vi "Set Actuator Voltage.vi"(6 "Enable":variant, 8 "error in (no error)":errorcluster, 9 "AO IOName Idx":i32, 10 "ActuatorV":dbl, 11 "DAQ":refnum<class "DAQ.lvclass">) -> (0 "error out":errorcluster, 3 "DAQ":refnum<class "DAQ.lvclass">)   [LabVIEW 2017, in "DAQ.lvclass"]
doc: "Developed by Kevin Thompson\nkevin@thompsonengineering.net\n\nCopyright 2015\nThompson Engineering, LLC"
uses:
  DAQ.lvclass
  DAQ.lvclass/DAQ.ctl
  Accessors/Get DAQ Settings.vi
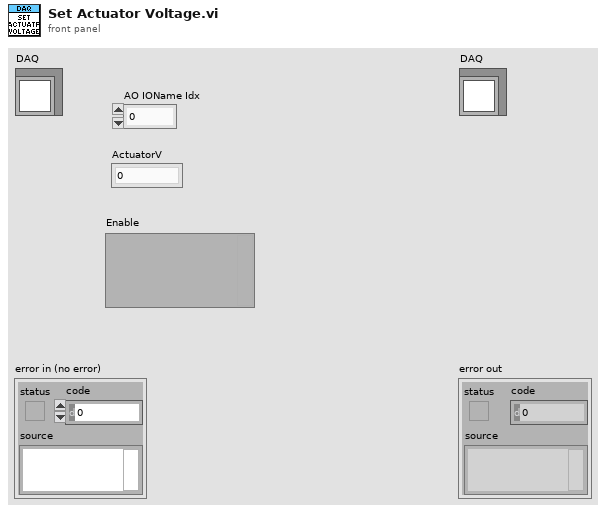
[diagram p1: front panel]
types:
  T1 = typedef "Type Descriptor Enumeration__ogtk.ctl" = enum8{"<Null>", "I8", "I16", "I32", "I64", "U8", "U16", "U32", "U64", "SGL", "DBL", "EXT", "CSG", "CDB", "CXT", "0x0F", "0x10", "0x11", "0x12", "0x13", "0x14", "Enum U8", "Enum U16", "Enum U32", "Enum U64", "SGL PQ", "DBL PQ", "EXT PQ", "CSG PQ", "CDB PQ", "CXT PQ", "0x1F", "0x20", "Boolean", "0x22", "0x23", "0x24", "0x25", "0x26", "0x27", "0x28", "0x29", "0x2A", "0x2B", "0x2C", "0x2D", "0x2E", "0x2F", "String", "0x31", "Path", "Pict", "0x34", "0x35", "0x36", "DAQ", "0x38", "0x39", "0x3A", "0x3B", "0x3C", "0x3D", "0x3E", "0x3F", "Array", "0x41", "0x42", "0x43", "0x44", "0x45", "0x46", "0x47", "0x48", "0x49", "0x4A", "0x4B", "0x4C", "0x4D", "0x4E", "0x4F", "Cluster", "0x51", "0x52", "Variant", "Waveform", "0x55", "0x56", "0x57", "0x58", "0x59", "0x5A", "0x5B", "0x5C", "0x5D", "0x5E", "0x5F", "0x60", "0x61", "0x62", "0x63", "0x64", "0x65", "0x66", "0x67", "0x68", "0x69", "0x6A", "0x6B", "0x6C", "0x6D", "0x6E", "0x6F", "Refnum"}
  T2 = typedef "DAQ.lvclass/TD DAQ Settings--cluster.ctl" = cluster{"Simulate DAQ":bool, "DI Settings":T3[], "AI Settings":T4[], "Relay IONames":string[], "AO IONames":string[], "AO NChan SingleTask":bool}
  T3 = typedef "DAQ.lvclass/TD DI Instrument Settings--cluster.ctl" = cluster{"Disable":bool, "DI TaskName":string, "DI RefreshIntv":i32}
  T4 = typedef "DAQ.lvclass/TD AI Instrument Settings--cluster.ctl" = cluster{"Disable":bool, "AI TaskName":string, "AI InstSettings":T5, "SimAI Ranges":T6}
  T5 = typedef "DAQ.lvclass/TD AI InstSettings--cluster.ctl" = cluster{"DaqRate":dbl, "NumSamples":i32}
  T6 = typedef "DAQ.lvclass/TD SimAI Ranges--cluster.ctl" = cluster{"lo":dbl, "hi":dbl}
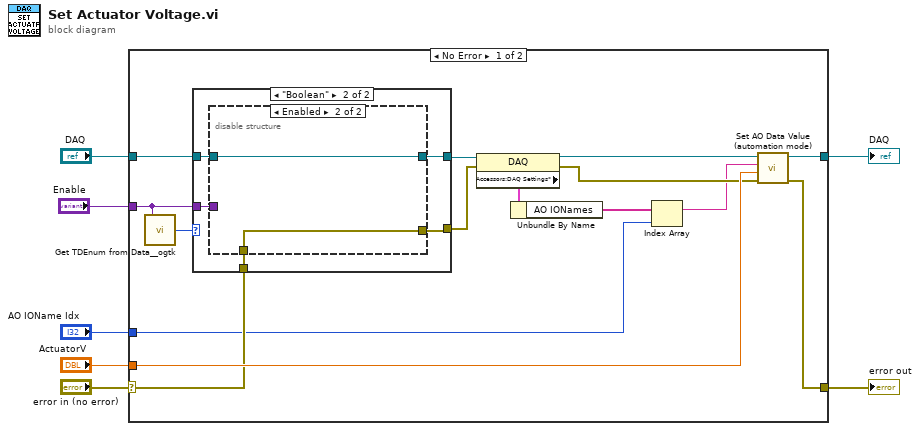
[diagram p0: block diagram]
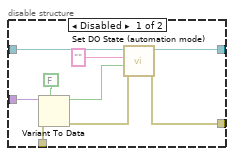
[diagram p3: hidden frame]
diagram:
  n1 = case shown="No Error" "error in (no error)" {
    selector: "error in (no error)" -> [w16 w42]
    tunnel: [w19 w42] -> w6
    tunnel: [w21 w41] -> w4
    tunnel: "DAQ" -> [w22 w41]
    tunnel: "Enable" -> [w17 _]
    tunnel: "ActuatorV" -> [w20 _]
    tunnel: "AO IOName Idx" -> [w8 _]
    frame No Error {
      n2 = call <userlib>:"Get TDEnum from Data__ogtk.vi"("Data"=w17) -> ("Type Descriptor Enumeration"=w18:T1)  [unwired: 4 in]
      n3 = case shown="\"Boolean\"" w18 {
        tunnel: w22 -> [w24 w29]
        tunnel: [w24 w28] -> w15
        tunnel: w17 -> [_ w27]
        tunnel: w16 -> [w23 w26]
        tunnel: [w23 w25] -> w13
        frame "<Null>", Default {
        }
        frame "Boolean" {
          n4 = disable-structure shown="Enabled" {
            disable-tunnel: w29 -> [w38 w40]
            disable-tunnel: [w37 w40] -> w28
            disable-tunnel: w27 -> [w36 _]
            disable-tunnel: w26 -> [w32 w39]
            disable-tunnel: [w31 w39] -> w25
            frame Disabled {
              n5 = Variant To Data(error in=w32, type=FALSE, Variant=w36) -> (data=w34:bool, error out=w33:errorcluster)
              n6 = call "Set DO State (automation mode).vi"("error in (no error)"=w33, "State"=w34, "DO IOName"="", "DAQ"=w38) -> ("error out"=w31:errorcluster, "DAQ"=w37:refnum<class "DAQ.lvclass">)  [unwired: 6 in]
            }
            frame Enabled {
            }
          }
        }
      }
      n7 = property class="DAQ"(reference=w15, error in=w13) -> (reference out=w14:refnum<class "DAQ.lvclass">, error out=w12:errorcluster, "Accessors:DAQ Settings*"=w11:T2)
      n8 = Unbundle By Name(w11) -> ("AO IONames"=w10:string[])
      n9 = Index Array(array=w10, index=w8) -> (element=w9:string)
      n10 = call "Set AO Data Value (automation mode).vi"("error in (no error)"=w12, "Value"=w20, "AO IOName"=w9, "DAQ"=w14) -> ("error out"=w19:errorcluster, "DAQ"=w21:refnum<class "DAQ.lvclass">)  [unwired: 6 in]
    }
    frame Error {
    }
  }
  "error out" <- w6
  "DAQ" <- w4
